vi "CheckWorkerError.vi"(8 "error in (no error)":errorcluster, 10 "timeout in ms (0)":i32, 11 "ResultProcessor in":refnum<class "ResultProcessor.lvclass">) -> (0 "error out":errorcluster, 2 "AsyncWorkerError":errorcluster, 3 "ResultProcessor out":refnum<class "ResultProcessor.lvclass">)   [LabVIEW 2015, in "ResultProcessor.lvclass"]
uses:
  ResultProcessor.lvclass
  ResultProcessor.lvclass/ResultProcessor.ctl
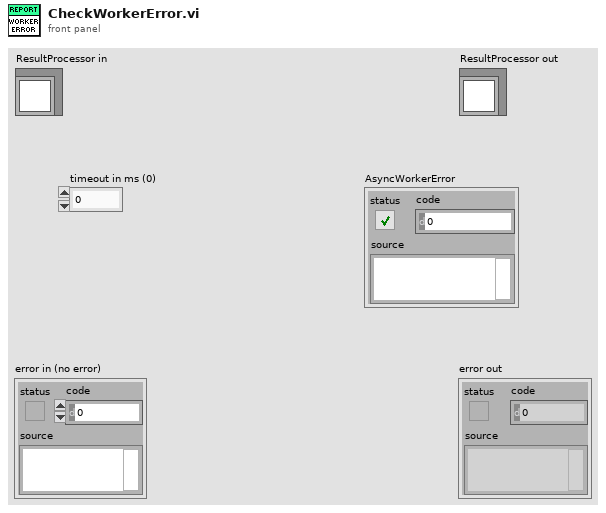
[diagram p1: front panel]
types:
  T1 = typedef "ResultProcessor.lvclass/ErrorQueueDataType.ctl" = cluster{"error out":errorcluster}
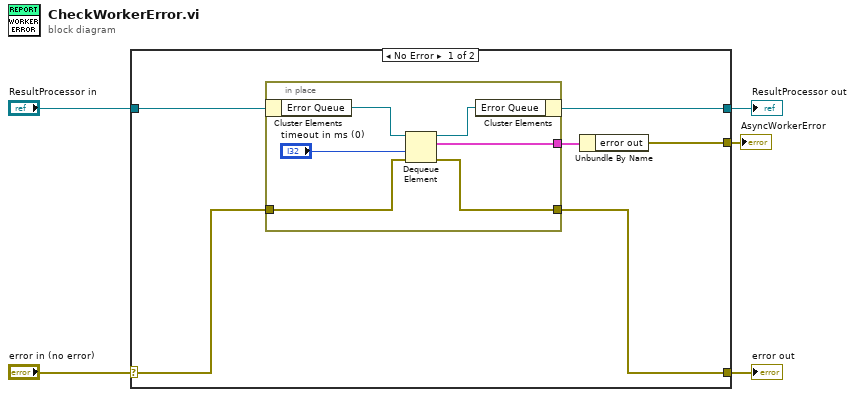
[diagram p0: block diagram]
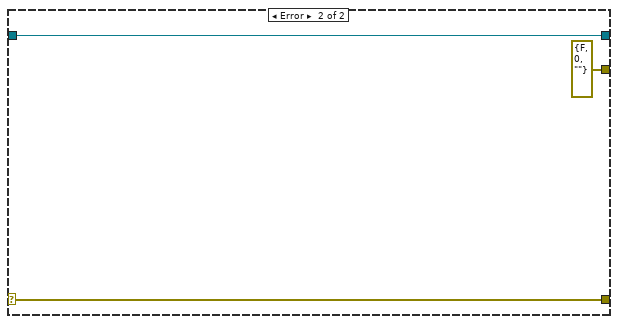
[diagram p2: hidden frame]
diagram:
  n1 = case shown="No Error" "error in (no error)" {
    selector: "error in (no error)" -> [w10 w20]
    tunnel: [w9 w20] -> w4
    tunnel: [w6 w19] -> w2
    tunnel: "ResultProcessor in" -> [w11 w19]
    tunnel: [w7 errorcluster {"status"=FALSE, "code"=0, "source"=""} ("error out")] -> w1
    frame No Error {
      n2 = in-place {
        in-place-border: w10 -> [w15]
        in-place-border: [w14] -> w9
        in-place-border: [w12] -> w8
        n3 = in-place-cluster #1(w11) -> ("Error Queue"=w17:refnum<queue>)
        n4 = Dequeue Element(queue=w17, timeout in ms (-1)="timeout in ms (0)", error in (no error)=w15) -> (queue out=w16:refnum<queue>, element=w12:T1, error out=w14:errorcluster)  [unwired: 1 out]
        n5 = in-place-cluster #1("Error Queue"=w16) -> (w6:refnum<class "ResultProcessor.lvclass">)
      }
      n6 = Unbundle By Name(w8) -> ("error out"=w7:errorcluster)
    }
    frame Error {
    }
  }
  "error out" <- w4
  "ResultProcessor out" <- w2
  "AsyncWorkerError" <- w1
